vi "Apply selectors to GObject and children.vi"(8 "Error in":errorcluster, 10 "Owning item selectors":string[](array[string]), 11 "GObject in":refnum<vi>) -> (0 "Error out":errorcluster)   [LabVIEW 2019, in "LSS.lvlib"]
uses:
  LSS.lvlib
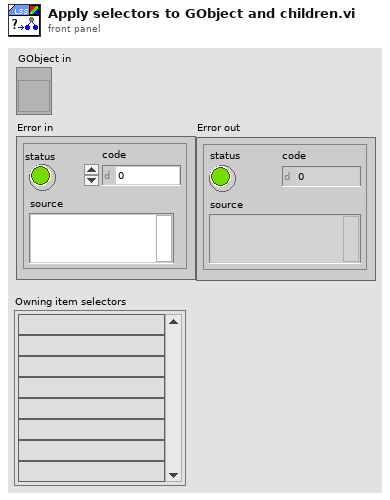
[diagram p1: front panel]
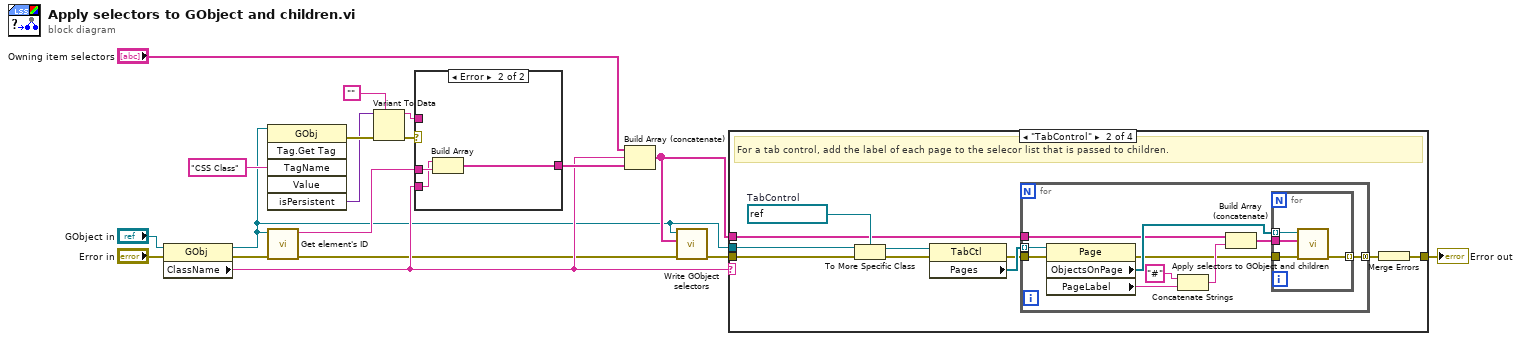
[diagram p0: block diagram]
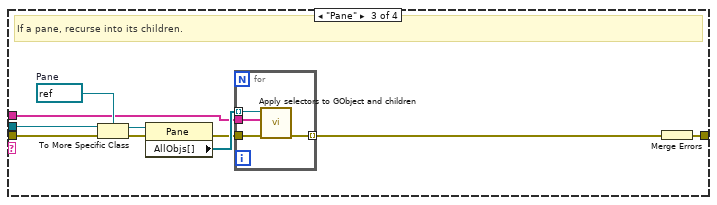
[diagram p3: hidden frame]
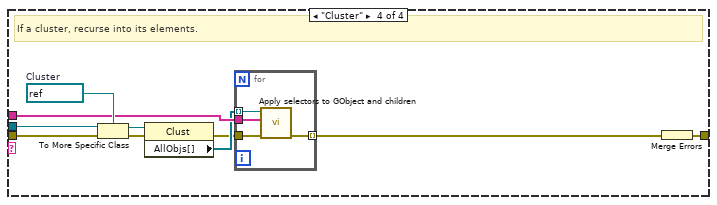
[diagram p4: hidden frame]
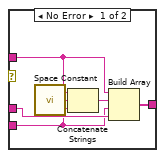
[diagram p5: hidden frame]
diagram:
  n1 = property class="GObj"(reference="GObject in", error in="Error in") -> (reference out=w1:refnum<vi>, error out=w5:errorcluster, "ClassName"=w7:string)
  n2 = invoke class="GObj" method="Tag.Get Tag"(reference=w1, "TagName"="CSS Class" ("Tag Name")) -> (error out=w11:errorcluster, "isPersistent"=w9:variant)  [unwired: 4 in, 4 out]
  n3 = call "Get element's ID.vi"("Error in"=w5, "GObject in"=w1) -> ("Error out"=w4:errorcluster, "ID"=w15:string)  [unwired: 8 in]
  n4 = Variant To Data(error in=w11, type="", Variant=w9) -> (data=w13:string, error out=w12:errorcluster)
  n5 = case shown="Error" w12 {
    tunnel: w15 -> [w22 w27]
    tunnel: w13 -> [w19 _]
    tunnel: [w24 w26] -> w14
    tunnel: w7 -> [w21 w25]
    frame No Error {
      n6 = call <vilib>:"Space Constant.vi"() -> ("String"=w23:string)
      n7 = Concatenate Strings(w19, w23, w21) -> (w20:string)
      n8 = Build Array(w19, w20, w21, w22) -> (w24:string[])
    }
    frame Error {
      n9 = Build Array(w25, w27) -> (w26:string[])
    }
  }
  n10 = Build Array (concatenate)("Owning item selectors", w7, w14) -> (w6:string[])
  n11 = call "Write GObject selectors.vi"("Error in"=w4, "Selectors"=w6, "GObject in"=w1) -> ("Error out"=w3:errorcluster)  [unwired: 8 in]
  n12 = case shown="\"TabControl\"" w7 {
    tunnel: w1 -> [_ w38 w62 w76]
    tunnel: w6 -> [_ w34 w53 w73]
    tunnel: w3 -> [w28 w31 w58 w69]
    tunnel: [w28 w32 w59 w70] -> w2
    frame Default {
    }
    frame "TabControl" {
      w37 = refnum<vi> refnum  # TabControl
      # "For a tab control, add the label of each page to the selecor list that is passed to children."
      n13 = To More Specific Class(target class=w37, reference=w38, error in=w31) -> (specific class reference=w36:refnum<vi>, error out=w30:errorcluster)
      n14 = property class="TabCtl"(reference=w36, error in=w30) -> (error out=w29:errorcluster, "Pages"=w35:refnum<vi>[])  [unwired: 1 out]
      n15 = for {
        tunnel: w35 -> [w48] mode=indexing
        tunnel: w34 -> [w45]
        tunnel: [w41] -> w33 mode=concatenating
        tunnel: w29 -> [w40]
        n16 = property class="Page"(reference=w48, error in=w40) -> (error out=w39:errorcluster, "ObjectsOnPage"=w47:refnum<vi>[], "PageLabel"=w46:string)  [unwired: 1 out]
        n17 = Concatenate Strings("#" ("string"), w46) -> (w43:string)
        n18 = Build Array (concatenate)(w45, w43) -> (w44:string[])
        n19 = for {
          tunnel: w47 -> [w52] mode=indexing
          tunnel: w44 -> [w51]
          tunnel: [w50] -> w41 mode=indexing
          tunnel: w39 -> [w49]
          n20 = call "Apply selectors to GObject and children.vi"("Error in"=w49, "Owning item selectors"=w51, "GObject in"=w52) -> ("Error out"=w50:errorcluster)  [unwired: 8 in]
        }
      }
      n21 = Merge Errors(w33) -> (w32:errorcluster)
    }
    frame "Pane" {
      w61 = refnum<vi> refnum  # Pane
      # "If a pane, recurse into its children."
      n22 = To More Specific Class(target class=w61, reference=w62, error in=w58) -> (specific class reference=w54:refnum<vi>, error out=w57:errorcluster)
      n23 = property class="Pane"(reference=w54, error in=w57) -> (error out=w55:errorcluster, "AllObjs[]"=w56:refnum<vi>[])  [unwired: 1 out]
      n24 = for {
        tunnel: w56 -> [w66] mode=indexing
        tunnel: w53 -> [w65]
        tunnel: [w64] -> w60 mode=indexing
        tunnel: w55 -> [w63]
        n25 = call "Apply selectors to GObject and children.vi"("Error in"=w63, "Owning item selectors"=w65, "GObject in"=w66) -> ("Error out"=w64:errorcluster)  [unwired: 8 in]
      }
      n26 = Merge Errors(w60) -> (w59:errorcluster)
    }
    frame "Cluster" {
      w75 = refnum<vi> refnum  # Cluster
      # "If a cluster, recurse into its elements."
      n27 = To More Specific Class(target class=w75, reference=w76, error in=w69) -> (specific class reference=w74:refnum<vi>, error out=w68:errorcluster)
      n28 = property class="Clust"(reference=w74, error in=w68) -> (error out=w67:errorcluster, "AllObjs[]"=w72:refnum<vi>[])  [unwired: 1 out]
      n29 = for {
        tunnel: w72 -> [w80] mode=indexing
        tunnel: w73 -> [w79]
        tunnel: w67 -> [w78]
        tunnel: [w77] -> w71 mode=indexing
        n30 = call "Apply selectors to GObject and children.vi"("Error in"=w78, "Owning item selectors"=w79, "GObject in"=w80) -> ("Error out"=w77:errorcluster)  [unwired: 8 in]
      }
      n31 = Merge Errors(w71) -> (w70:errorcluster)
    }
  }
  "Error out" <- w2
